vi "autofocus-view-calibration.vi"(10 "stop":bool, 11 "?":bool) -> (0 "Intensity 2":cluster{"X position":dbl, "Y position":dbl}(graph), 1 "Power Intensity":dbl(graph), 2 "Calibration curve":cluster{ext[], dbl[]}(graph), 3 "XY Position":cluster{"Y":dbl[], "Y":dbl[]}[](graph)=[{"Y"=[30.68], "Y"=[27.36]}])   [LabVIEW 2014]
uses:
  autofocus-globals.vi
  tirf-lock-globals.vi
panel:
  in  "Shutter Camera \nduring calibration?":bool
  in  "Display":bool=TRUE
  # "Divide \nBy Sum"
  # "Raw"
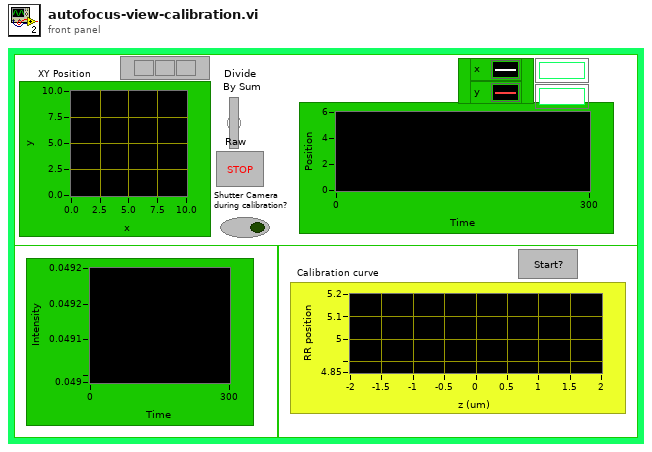
[diagram p1: front panel]
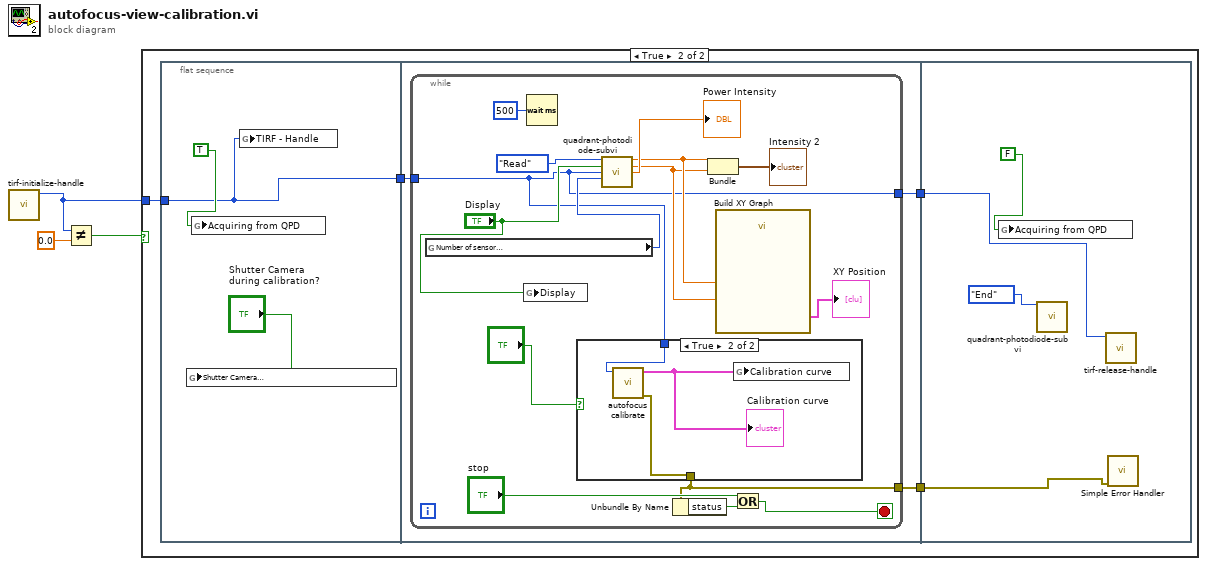
[diagram p0: block diagram]
diagram:
  n1 = call "tirf-initialize-handle.vi"() -> ("handle"=w1:i32)  [unwired: 11 in]
  n2 = Not Equal?(x=w1, y=0.0) -> (x != y?=w2:bool)
  n3 = case shown="True" w2 {
    tunnel: w1 -> [_ w5]
    frame False {
    }
    frame True {
      n4 = flat-sequence {
        tunnel: [w9] -> w6
        tunnel: w5 -> [w9]
        tunnel: [w13] -> w7
        tunnel: w6 -> [w12]
        tunnel: [w11] -> w4
        tunnel: w7 -> [w32]
        tunnel: w4 -> [w33]
        frame #0 {
          n5 = global write "autofocus-globals.vi" "Shutter Camera\nduring calibration?"("Shutter Camera \nduring calibration?") -> ()
          n6 = global write "autofocus-globals.vi" "Acquiring from QPD"(TRUE) -> ()
          n7 = global write "autofocus-globals.vi" "TIRF - Handle"(w9) -> ()
        }
        frame #1 {
          n8 = while {
            tunnel: [w17] -> w13
            tunnel: w12 -> [w14]
            tunnel: [w14] -> w11
            stop <- w18 stop-if-true
            n9 = global read "autofocus-globals.vi" "Number of sensor\nreadings to average"() -> (w16:i32)
            n10 = global write "tirf-lock-globals.vi" "Display"("Display") -> ()
            n11 = Wait (ms)(milliseconds to wait=u32 500) -> ()  [unwired: 1 out]
            n12 = case shown="True" "?" {
              tunnel: [_ w30] -> w17
              tunnel: w14 -> [_ w29]
              frame False {
              }
              frame True {
                n13 = call "autofocus calibrate.vi"("Handle"=w29) -> ("Error Out"=w30:errorcluster, "Cal. curve"=w31:cluster{ext[], dbl[]})  [unwired: 8 in, 1 out]
                "Calibration curve" <- w31
                n14 = global write "autofocus-globals.vi" "Calibration curve"(w31) -> ()
              }
            }
            n15 = call "quadrant-photodiode-subvi.vi"("Mode"=enum16{"Start", "Read", "End"}."Read", "Display"="Display", "Handle"=w14, "Averages"=w16) -> ("coerced(x)"=w24:dbl, "coerced(y)"=w23:dbl, "Power (mw)"=→"Power Intensity":dbl)  [unwired: 9 in]
            n16 = Unbundle By Name(w17) -> ("status"=w19:bool)
            n17 = Bundle("coerced(x)"=w24, "coerced(y)"=w23) -> (→"Intensity 2":cluster{"coerced(x)":dbl, "coerced(y)":dbl})  [unwired: 1 in]
            n18 = call "Build XY Graph"("Y Input"=w23, "X Input"=w24) -> ("XY Graph"=→"XY Position":cluster{"Y":dbl[], "Y":dbl[]}[])  [unwired: 3 in, 6 out]
            n19 = Or(x="stop", y=w19) -> (x .or. y?=w18:bool)
          }
        }
        frame #2 {
          n20 = global write "autofocus-globals.vi" "Acquiring from QPD"(FALSE) -> ()
          n21 = call "quadrant-photodiode-subvi.vi"("Mode"=enum16{"Start", "Read", "End"}."End") -> ()  [unwired: 12 in, 3 out]
          n22 = call "tirf-release-handle.vi"("handle"=w33) -> ()  [unwired: 11 in]
          n23 = call <vilib>:"Simple Error Handler.vi"("error in (no error)"=w32) -> ()  [unwired: 1 in, 8 out]
        }
      }
    }
  }
